vi "glsl_set_spots_string.vi"(5 "spots uniforms":i32[](array[numeric])=[2, 13, 15, 17], 6 "Use Textures?":bool, 7 "n uniforms":i32[](array[numeric])=[0, 12, 14, 16], 10 "Spots (2D Array)":dbl[][](array[numeric]), 11 "Preceding String":string) -> (3 "Uniform-Setting String":string)   [LabVIEW 2010]
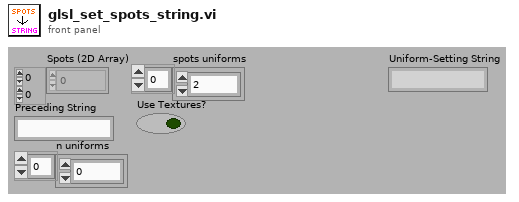
[diagram p1: front panel]
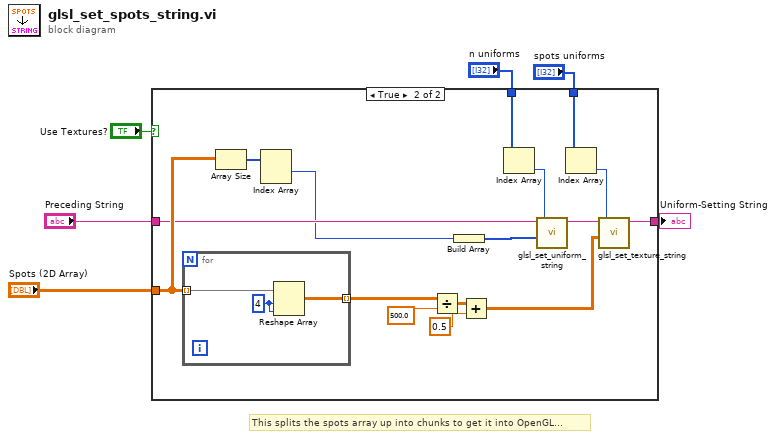
[diagram p0: block diagram]
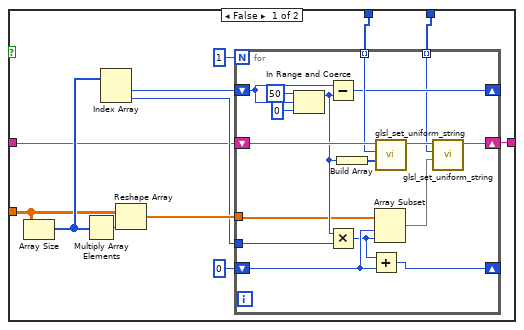
[diagram p2: hidden frame]
diagram:
  # "This splits the spots array up into chunks to get it into OpenGL..."
  n1 = case shown="True" "Use Textures?" {
    tunnel: "n uniforms" -> [w9 w51]
    tunnel: "spots uniforms" -> [w8 w50]
    tunnel: "Spots (2D Array)" -> [w10 w49]
    tunnel: "Preceding String" -> [w11 w48]
    tunnel: [w7 w47] -> w2
    frame False {
      n2 = Array Size(array=w10) -> (size(s)=w13:i32[])
      n3 = Multiply Array Elements(1:w13) -> (0:w18:i32)
      n4 = Index Array(array=w13) -> (element #1=w15:i32, element #2=w14:i32)  [unwired: 2 in]
      n5 = Reshape Array(w10, w18) -> (w16:dbl[])
      n6 = for {
        N: 1 -> [_]
        shift-right: [w23] -> w7
        shift-left: w11 -> [w34]
        tunnel: w9 -> [w33] mode=indexing
        shift-right: [w29] -> _
        shift-left: w15 -> [w30]
        tunnel: w16 -> [w27]
        shift-right: [w24] -> _
        shift-left: 0 -> [w26]
        tunnel: w8 -> [w21] mode=indexing
        tunnel: w14 -> [w19]
        n7 = In Range and Coerce(upper limit=50, x=w30, lower limit=0) -> (coerced(x)=w28:i32)  [unwired: 1 out]
        n8 = Subtract(x=w30, y=w28) -> (x-y=w29:i32)
        n9 = Multiply(x=w28, y=w19) -> (x*y=w25:i32)
        n10 = Build Array(w28) -> (w35:i32[])
        n11 = Add(x=w25, y=w26) -> (x+y=w24:i32)
        n12 = Array Subset(array=w27, index=w26, length=w25) -> (w20:dbl[])
        n13 = call "glsl_set_uniform_string.vi"("Uniform Value"=w35, "uniform index"=w33, "initial string"=w34) -> ("Uniform-setting string"=w22:string)  [unwired: 3 in, 1 out]
        n14 = call "glsl_set_uniform_string.vi"("Uniform Value"=w20, "uniform index"=w21, "initial string"=w22) -> ("Uniform-setting string"=w23:string)  [unwired: 3 in, 1 out]
      }
    }
    frame True {
      n15 = for {
        tunnel: w49 -> [w54] mode=indexing
        tunnel: [w52] -> w40 mode=indexing
        w53 = 4 ("dimension size")
        n16 = Reshape Array(w54, w53, w53) -> (w52:dbl[][])
      }
      n17 = Array Size(array=w49) -> (size(s)=w45:i32[])
      n18 = Index Array(array=w45) -> (element #1=w42:i32)  [unwired: 2 in, 1 out]
      n19 = Divide(x=w40, y=500.0 ("dimension size")) -> (x/y=w38:dbl[][][])
      n20 = Build Array(w42) -> (w41:i32[])
      n21 = Add(x=w38, y=0.5 ("dimension size")) -> (x+y=w36:dbl[][][])
      n22 = Index Array(array=w51) -> (element=w43:i32)  [unwired: 1 in]
      n23 = call "glsl_set_uniform_string.vi"("Uniform Value"=w41, "uniform index"=w43, "initial string"=w48) -> ("Uniform-setting string"=w44:string)  [unwired: 3 in, 1 out]
      n24 = Index Array(array=w50) -> (element=w46:i32)  [unwired: 1 in]
      n25 = call "glsl_set_texture_string.vi"("Uniform Value"=w36, "uniform index"=w46, "initial string"=w44) -> ("Uniform-setting string"=w47:string)  [unwired: 4 in]
    }
  }
  "Uniform-Setting String" <- w2
